vi "Ev Data Path.vi"(8 "error in (no error)":errorcluster, 11 "Pic Json Generator in":refnum<class "Pic Json Generator.lvclass">) -> (0 "error out":errorcluster, 3 "Pic Json Generator out":refnum<class "Pic Json Generator.lvclass">)   [LabVIEW 2018, in "Pic Json Generator.lvlib" / "Pic Json Generator.lvclass"]
uses:
  Pic Json Generator.lvclass
  Pic Json Generator.lvclass/Pic Json Generator.ctl
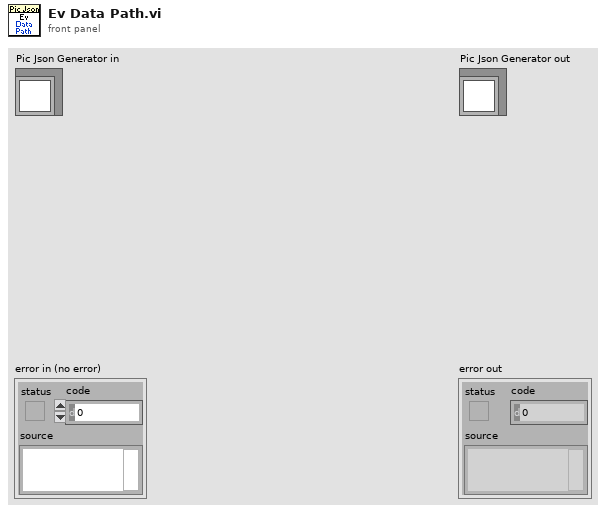
[diagram p1: front panel]
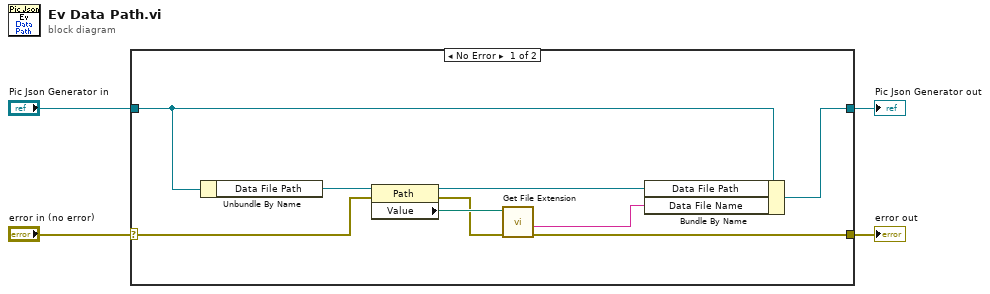
[diagram p0: block diagram]
diagram:
  n1 = case shown="No Error" "error in (no error)" {
    selector: "error in (no error)" -> [w11 w15]
    tunnel: [w8 w15] -> w3
    tunnel: [w7 w14] -> w1
    tunnel: "Pic Json Generator in" -> [w13 w14]
    frame No Error {
      n2 = Unbundle By Name(w13) -> ("Data File Path"=w12:refnum<vi>)
      n3 = property class="Path"(reference=w12, error in=w11) -> (reference out=w5:refnum<vi>, error out=w9:errorcluster, "Value"=w10:path)
      n4 = call <vilib>:"Get File Extension.vi"("error in (no error)"=w9, "file"=w10) -> ("error out"=w8:errorcluster, "filename without extension"=w6:string)  [unwired: 5 in, 3 out]
      n5 = Bundle By Name(cluster=w13, "Data File Path"=w5, "Data File Name"=w6) -> (w7:refnum<class "Pic Json Generator.lvclass">)
    }
    frame Error {
    }
  }
  "error out" <- w3
  "Pic Json Generator out" <- w1
